vi "Bscan.vi"() -> ()   [LabVIEW 2017]
panel:
  out "B [mT]":dbl[](array[numeric])
  in  "z":dbl
  in  "y":dbl
  in  "x":dbl
  in  "directory name":string="D:\\LabView\\Data\\MetroLab\\"
  out "output text":string
  in  "error in (no error)":errorcluster caption="エラー入力（エラーなし）"
  out "error out":errorcluster caption="エラー出力" {"code" format="%.0x"}
  in  "filename":string="Bscan.txt"
  # "Position"
  # "x"
  # "y"
  # "z"
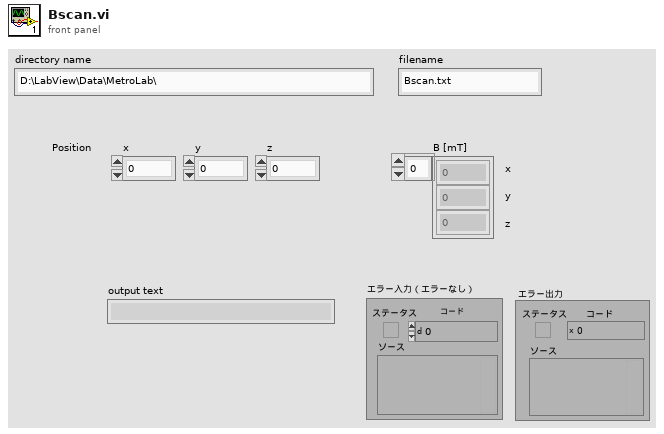
[diagram p1: front panel]
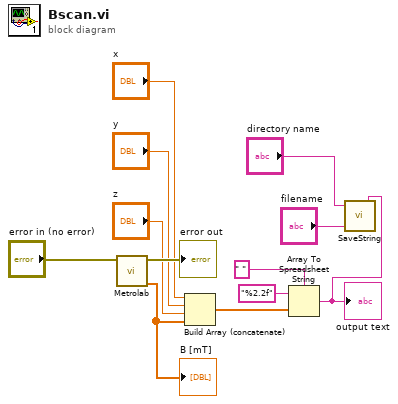
[diagram p0: block diagram]
diagram:
  n1 = call "Metrolab.vi"("error in (no error)"="error in (no error)") -> ("配列"=w1:dbl[], "error out"=→"error out":errorcluster)  [unwired: 5 in]
  "B [mT]" <- w1
  n2 = Build Array (concatenate)("x", "y", "z", w1) -> (w2:dbl[])
  n3 = Array To Spreadsheet String(delimiter (Tab)=" " ("デリミタ（'\\'コード表示）"), array=w2, 3:"%2.2f" ("形式文字列")) -> (spreadsheet string=w8:string)
  "output text" <- w8
  n4 = call "SaveString.vi"("input string"=w8, "filename"="filename", "directory name"="directory name") -> ()  [unwired: 3 in]
